vi "Main.vi"() -> ()   [LabVIEW 2018] (continued)
            n1595 = Concatenate Strings("Where QRCode='" ("查询语句"), w1146, "'" ("字符串")) -> (w1171:string)
            n1596 = call "SQL_Select.vi"("要读取的列名"=string[] ["Last_Station", "Last_Result"], "表名"="Online", "error in (no error)"=w1177, "查询语句"=w1171, "查询条件"=TRUE, "connection reference"=w1178) -> ("error out"=w1150:errorcluster, "数据"=w1170:string[][])  [unwired: 3 in, 1 out]
            n1597 = case shown="无错误" w1150 {
              tunnel: w1170 -> [w1185 _]
              tunnel: ["1" ("右扫码请求回复") "2" ("右扫码请求回复")] -> w1162
              tunnel: [w1180 w1186] -> w1161
              tunnel: [w1179 w1186] -> w1160
              frame No Error {
                n1598 = Index Array(array=w1185, index (row)=0 ("索引 (行)")) -> (element=w1182:string[])  [unwired: 1 in]
                n1599 = Index Array(array=w1182, index #1=0 ("索引 (行)")) -> (element #1=w1180:string, element #2=w1179:string)  [unwired: 1 in]
                "上一站号(102)" <- w1180
                "上一站结果(102)" <- w1179
              }
              frame Error {
                w1186 = ""
              }
            }
            n1600 = Insert Into Array(array=string[] [] ("数组"), index=0 ("索引"), new element #1=w1162, new element #2=w1161, new element #3=w1160) -> (w1167:string[])
            n1601 = Format Date/Time String(time format string (%c)="%Y-%m-%d" ("时间格式字符串(%c)")) -> (date/time string=w1158:string)  [unwired: 2 in]
            n1602 = Get Date/Time String() -> (time string=w1157:string)  [unwired: 3 in, 1 out]
            n1603 = Bundle By Name(cluster=cluster{"Data":string[], "State":T1} {"Data"=[], "State"=enum."PLC通讯初始化"} ("元素"), "Data"=w1167, "State"=状态2."扫码回复2") -> (w1168:cluster{"Data":string[], "State":T1})
            n1604 = Enqueue Element(queue=w1163, element=w1168) -> ()  [unwired: 2 in, 3 out]
            n1605 = Insert Into Array(array=string[] [] ("数组"), index=0 ("索引"), new element #1=w1158, new element #2=w1157, new element #3=w1146) -> (w1154:string[])
            n1606 = Insert Into Array(array=string[][] [] ("数组"), index (row)=0 ("索引 (行)"), new element=w1154) -> (w1151:string[][])  [unwired: 1 in]
            n1607 = Transpose 2D Array(2D array=w1151) -> (transposed array=w1148:string[][])
            n1608 = property on="ST10-2_DATA" class="MCListbox (严格)"("ItemNames"=w1148) -> ()  [unwired: 2 in, 2 out]
          }
          event "ST102数据读取（事件）": Value Change {
            w1211 = 0 ("索引 (行)")
            n1609 = event-data() -> ()  [unwired: 1 in, 2 out]
            n1610 = local read "102读取数据"() -> (w1188:string[])
            n1611 = local read "102 二维码"() -> (w1193:string)
            n1612 = Concatenate Strings("Where QRCode='" ("查询语句"), w1193, "'" ("字符串")) -> (w1218:string)
            n1613 = call "SQL_Select.vi"("要读取的列名"=string[] ["Rework_Status"], "表名"="Online", "error in (no error)"=w1195, "查询语句"=w1218, "查询条件"=TRUE, "connection reference"=w1196) -> ("error out"=w1213:errorcluster, "数据"=w1217:string[][], "connection reference out"=w1214:T12)  [unwired: 3 in]
            n1614 = Index Array(array=w1217, index (row)=w1211, index (col)=w1211) -> (element=w1216:string)
            n1615 = Equal?(x=w1216, y="T") -> (x = y?=w1215:bool)
            n1616 = case shown="真" w1215 {
              tunnel: [w1235 w1241] -> w1223
              tunnel: w1188 -> [w1234 w1244]
              tunnel: [w1229 w1240] -> w1191
              tunnel: w1193 -> [w1228 w1243]
              tunnel: w1218 -> [w1227 w1242]
              tunnel: w1214 -> [w1226 w1255]
              tunnel: w1213 -> [w1225 w1254]
              frame False {
                n1617 = call "SQL_Update.vi"("查询语句"=w1227, "表名"="Online", "error in (no error)"=w1225, "列名对应的值"=w1234, "列名"=string[] ["Last_Station", "Last_Result", "ST102_Date", "ST102_Time", "ST102_Package_Result"], "connection reference"=w1226) -> ("error out"=w1229:errorcluster)  [unwired: 4 in, 1 out]
                n1618 = Unbundle By Name(w1229) -> ("status"=w1233:bool)
                n1619 = Equal?(x=w1228, y="") -> (x = y?=w1231:bool)
                n1620 = Or(x=w1233, y=w1231) -> (x .or. y?=w1230:bool)
                n1621 = case shown="假" w1230 {
                  tunnel: ["1" ("数据保存请求回复") "2" ("数据保存请求回复")] -> w1235
                  frame False {
                  }
                  frame True {
                  }
                }
              }
              frame True {
                w1250 = 0 ("索引 (行)")
                n1622 = call "SQL_Select.vi"("要读取的列名"=string[] ["[102]"], "表名"="Rework_List", "error in (no error)"=w1254, "查询语句"=w1242, "查询条件"=TRUE, "connection reference"=w1255) -> ("error out"=w1245:errorcluster, "数据"=w1251:string[][], "connection reference out"=w1246:T12)  [unwired: 3 in]
                n1623 = Index Array(array=w1251, index (row)=w1250, index (col)=w1250) -> (element=w1249:string)
                n1624 = Equal?(x=w1249, y="T") -> (x = y?=w1247:bool)
                n1625 = case shown="真" w1247 {
                  tunnel: w1246 -> [w1263 w1282]
                  tunnel: w1245 -> [w1264 w1281]
                  tunnel: w1244 -> [w1262 w1288]
                  tunnel: w1243 -> [w1259 w1283]
                  tunnel: w1242 -> [w1261 w1275]
                  tunnel: [w1258 w1274] -> w1241
                  tunnel: [w1260 w1273] -> w1240
                  frame False {
                    n1626 = call "SQL_Update.vi"("查询语句"=w1261, "表名"="Online", "error in (no error)"=w1264, "列名对应的值"=w1262, "列名"=string[] ["Last_Station", "Last_Result", "ST101_Date", "ST101_Time", "ST101_Package_Result", "ST101_Shaft_M0102049", "ST101_Form_Seal_5026859", "ST101_Dowel_Pin_5024532", "ST101_Dowel_Pin_5020281", "ST101_Control_Plat_5025303", "ST101_Flange_M0104918"], "connection reference"=w1263) -> ("error out"=w1260:errorcluster)  [unwired: 4 in, 1 out]
                    n1627 = Unbundle By Name(w1260) -> ("status"=w1268:bool)
                    n1628 = Equal?(x=w1259, y="") -> (x = y?=w1266:bool)
                    n1629 = Or(x=w1268, y=w1266) -> (x .or. y?=w1265:bool)
                    n1630 = case shown="假" w1265 {
                      tunnel: ["1" ("数据保存请求回复") "2" ("数据保存请求回复")] -> w1258
                      frame False {
                      }
                      frame True {
                      }
                    }
                  }
                  frame True {
                    n1631 = Delete From Array(array=w1288, length=2 ("长度"), index=0 ("索引")) -> (deleted portion=w1276:string[], array with subset deleted=w1285:string[])
                    n1632 = call "SQL_Update.vi"("查询语句"=w1275, "表名"="Online", "error in (no error)"=w1281, "列名对应的值"=w1276, "列名"=string[] ["Last_Station", "Last_Result"], "connection reference"=w1282) -> ("error out"=w1280:errorcluster, "connection reference 2"=w1279:T12)  [unwired: 4 in]
                    n1633 = call "SQL_Update.vi"("查询语句"=w1275, "表名"="Rework", "error in (no error)"=w1280, "列名对应的值"=w1285, "列名"=string[] ["ST102_Date", "ST102_Time", "ST102_Package_Result"], "connection reference"=w1279) -> ("error out"=w1273:errorcluster)  [unwired: 4 in, 1 out]
                    n1634 = Unbundle By Name(w1273) -> ("status"=w1291:bool)
                    n1635 = Equal?(x="", y=w1283) -> (x = y?=w1290:bool)
                    n1636 = Or(x=w1291, y=w1290) -> (x .or. y?=w1289:bool)
                    n1637 = case shown="假" w1289 {
                      tunnel: ["1" ("数据保存请求回复") "2" ("数据保存请求回复")] -> w1274
                      frame False {
                      }
                      frame True {
                      }
                    }
                  }
                }
              }
            }
            n1638 = Insert Into Array(array=string[] [] ("数组"), index=0 ("索引"), new element=w1223) -> (w1224:string[])
            n1639 = Delete From Array(array=w1188, length=2 ("长度"), index=0 ("索引")) -> (array with subset deleted=w1220:string[])  [unwired: 1 out]
            n1640 = Bundle By Name(cluster=cluster{"Data":string[], "State":T1} {"Data"=[], "State"=enum."PLC通讯初始化"} ("元素"), "Data"=w1224, "State"=状态2."数据保存回复2") -> (w1222:cluster{"Data":string[], "State":T1})
            n1641 = Insert Into Array(array=w1220, index=2 ("索引"), new element=w1193) -> (w1219:string[])
            n1642 = Enqueue Element(queue=w1194, element=w1222) -> ()  [unwired: 2 in, 3 out]
            n1643 = Insert Into Array(array=string[][] [] ("数组"), index (row)=0 ("索引 (行)"), new element=w1219) -> (w1221:string[][])  [unwired: 1 in]
            n1644 = Transpose 2D Array(2D array=w1221) -> (transposed array=w1192:string[][])
            n1645 = property on="ST10-2_DATA" class="MCListbox (严格)"("ItemNames"=w1192) -> ()  [unwired: 2 in, 2 out]
            "ST102数据读取（事件）" <- FALSE ("ST102数据读取（事件）")
          }
          event "ST202扫码请求(事件)": Value Change {
            n1646 = event-data() -> ()  [unwired: 1 in, 1 out]
            n1647 = local read "201二维码"() -> (w1295:string)
            n1648 = Concatenate Strings("Where QRCode='" ("查询语句"), w1295, "'" ("字符串")) -> (w1321:string)
            n1649 = call "SQL_Select.vi"("要读取的列名"=string[] ["Last_Station", "Last_Result"], "表名"="Online", "error in (no error)"=w1301, "查询语句"=w1321, "查询条件"=TRUE, "connection reference"=w1300) -> ("error out"=w1297:errorcluster, "数据"=w1320:string[][])  [unwired: 3 in, 1 out]
            n1650 = case shown="无错误" w1297 {
              tunnel: w1320 -> [w1334 _]
              tunnel: ["1" ("右扫码请求回复") "2" ("右扫码请求回复")] -> w1313
              tunnel: [w1329 w1335] -> w1312
              tunnel: [w1328 w1335] -> w1311
              frame No Error {
                n1651 = Index Array(array=w1334, index (row)=0 ("索引 (行)")) -> (element=w1331:string[])  [unwired: 1 in]
                n1652 = Index Array(array=w1331, index #1=0 ("索引 (行)")) -> (element #1=w1329:string, element #2=w1328:string)  [unwired: 1 in]
                "上一站号 (202)" <- w1329
                "上一站结果 (202)" <- w1328
              }
              frame Error {
                w1335 = ""
              }
            }
            n1653 = Insert Into Array(array=string[] [] ("数组"), index=0 ("索引"), new element #1=w1313, new element #2=w1312, new element #3=w1311) -> (w1317:string[])
            n1654 = Format Date/Time String(time format string (%c)="%Y-%m-%d" ("时间格式字符串(%c)")) -> (date/time string=w1309:string)  [unwired: 2 in]
            n1655 = Get Date/Time String() -> (time string=w1308:string)  [unwired: 3 in, 1 out]
            n1656 = Bundle By Name(cluster=cluster{"Data":string[], "State":T1} {"Data"=[], "State"=enum."PLC通讯初始化"} ("元素"), "Data"=w1317, "State"=状态2."扫码回复") -> (w1318:cluster{"Data":string[], "State":T1})
            n1657 = Insert Into Array(array=string[] [] ("数组"), index=0 ("索引"), new element #1=w1309, new element #2=w1308, new element #3=w1295) -> (w1305:string[])
            n1658 = Enqueue Element(queue=w1299, element=w1318) -> ()  [unwired: 2 in, 3 out]
            n1659 = Insert Into Array(array=string[][] [] ("数组"), index (row)=0 ("索引 (行)"), new element=w1305) -> (w1302:string[][])  [unwired: 1 in]
            n1660 = Transpose 2D Array(2D array=w1302) -> (transposed array=w1298:string[][])
            n1661 = property on="ST20-2_DATA" class="MCListbox (严格)"("ItemNames"=w1298) -> ()  [unwired: 2 in, 2 out]
            "ST202扫码请求(事件)" <- FALSE ("ST20扫码请求(事件)")
          }
          event "ST202数据读取(事件)": Value Change {
            w1349 = 0 ("索引 (行)")
            n1662 = event-data() -> ()  [unwired: 1 in, 1 out]
            n1663 = local read "201二维码"() -> (w1338:string)
            n1664 = local write "ST202数据读取(事件)"(FALSE ("ST20数据读取(事件)")) -> ()
            n1665 = Dequeue Element(queue=w1369, timeout in ms (-1)=10 ("超时毫秒(-1)")) -> (element=w1339:string[])  [unwired: 1 in, 3 out]
            n1666 = Concatenate Strings("Where QRCode='" ("查询语句"), w1338, "'" ("字符串")) -> (w1351:string)
            n1667 = call "SQL_Select.vi"("要读取的列名"=string[] ["Rework_Status"], "表名"="Online", "error in (no error)"=w1342, "查询语句"=w1351, "查询条件"=TRUE, "connection reference"=w1343) -> ("error out"=w1344:errorcluster, "数据"=w1350:string[][], "connection reference out"=w1345:T12)  [unwired: 3 in]
            n1668 = Index Array(array=w1350, index (row)=w1349, index (col)=w1349) -> (element=w1348:string)
            n1669 = Equal?(x=w1348, y="T") -> (x = y?=w1346:bool)
            n1670 = case shown="真" w1346 {
              tunnel: [w1387 w1392] -> w1340
              tunnel: w1339 -> [w1376 w1395]
              tunnel: [w1382 w1391] -> w1341
              tunnel: w1338 -> [w1381 w1394]
              tunnel: w1351 -> [w1380 w1393]
              tunnel: w1345 -> [w1379 w1406]
              tunnel: w1344 -> [w1378 w1405]
              frame False {
                n1671 = call "SQL_Update.vi"("查询语句"=w1380, "表名"="Online", "error in (no error)"=w1378, "列名对应的值"=w1376, "列名"=string[] ["Last_Station", "Last_Result", "ST202_Date", "ST202_Time", "ST202_Package_Result", "ST202_Rotor_5025805", "ST202_Camring_5026187", "ST202_Dowel_Pin_M0104893"], "connection reference"=w1379) -> ("error out"=w1382:errorcluster)  [unwired: 4 in, 1 out]
                n1672 = Unbundle By Name(w1382) -> ("status"=w1386:bool)
                n1673 = Equal?(x=w1381, y="") -> (x = y?=w1384:bool)
                n1674 = Or(x=w1386, y=w1384) -> (x .or. y?=w1383:bool)
                n1675 = case shown="假" w1383 {
                  tunnel: ["1" ("数据保存请求回复") "2" ("数据保存请求回复")] -> w1387
                  frame False {
                  }
                  frame True {
                  }
                }
              }
              frame True {
                w1401 = 0 ("索引 (行)")
                n1676 = call "SQL_Select.vi"("要读取的列名"=string[] ["[202]"], "表名"="Rework_List", "error in (no error)"=w1405, "查询语句"=w1393, "查询条件"=TRUE, "connection reference"=w1406) -> ("error out"=w1396:errorcluster, "数据"=w1402:string[][], "connection reference out"=w1397:T12)  [unwired: 3 in]
                n1677 = Index Array(array=w1402, index (row)=w1401, index (col)=w1401) -> (element=w1400:string)
                n1678 = Equal?(x=w1400, y="T") -> (x = y?=w1398:bool)
                n1679 = case shown="真" w1398 {
                  tunnel: w1397 -> [w1414 w1433]
                  tunnel: w1396 -> [w1415 w1432]
                  tunnel: w1395 -> [w1413 w1439]
                  tunnel: w1394 -> [w1410 w1434]
                  tunnel: w1393 -> [w1412 w1424]
                  tunnel: [w1409 w1426] -> w1392
                  tunnel: [w1411 w1425] -> w1391
                  frame False {
                    n1680 = call "SQL_Update.vi"("查询语句"=w1412, "表名"="Online", "error in (no error)"=w1415, "列名对应的值"=w1413, "列名"=string[] ["Last_Station", "Last_Result", "ST202_Date", "ST202_Time", "ST202_Package_Result", "ST202_Rotor_5025805", "ST202_Camring_5026187", "ST202_Dowel_Pin_M0104893"], "connection reference"=w1414) -> ("error out"=w1411:errorcluster)  [unwired: 4 in, 1 out]
                    n1681 = Unbundle By Name(w1411) -> ("status"=w1419:bool)
                    n1682 = Equal?(x=w1410, y="") -> (x = y?=w1417:bool)
                    n1683 = Or(x=w1419, y=w1417) -> (x .or. y?=w1416:bool)
                    n1684 = case shown="假" w1416 {
                      tunnel: ["1" ("数据保存请求回复") "2" ("数据保存请求回复")] -> w1409
                      frame False {
                      }
                      frame True {
                      }
                    }
                  }
                  frame True {
                    n1685 = Delete From Array(array=w1439, length=2 ("长度"), index=0 ("索引")) -> (deleted portion=w1427:string[], array with subset deleted=w1436:string[])
                    n1686 = call "SQL_Update.vi"("查询语句"=w1424, "表名"="Online", "error in (no error)"=w1432, "列名对应的值"=w1427, "列名"=string[] ["Last_Station", "Last_Result"], "connection reference"=w1433) -> ("error out"=w1431:errorcluster, "connection reference 2"=w1430:T12)  [unwired: 4 in]
                    n1687 = call "SQL_Update.vi"("查询语句"=w1424, "表名"="Rework", "error in (no error)"=w1431, "列名对应的值"=w1436, "列名"=string[] ["ST202_Date", "ST202_Time", "ST202_Package_Result", "ST202_Rotor_5025805", "ST202_Camring_5026187", "ST202_Dowel_Pin_M0104893"], "connection reference"=w1430) -> ("error out"=w1425:errorcluster)  [unwired: 4 in, 1 out]
                    n1688 = Unbundle By Name(w1425) -> ("status"=w1442:bool)
                    n1689 = Equal?(x="", y=w1434) -> (x = y?=w1441:bool)
                    n1690 = Or(x=w1442, y=w1441) -> (x .or. y?=w1440:bool)
                    n1691 = case shown="真" w1440 {
                      tunnel: ["1" ("数据保存请求回复") "2" ("数据保存请求回复")] -> w1426
                      frame False {
                      }
                      frame True {
                      }
                    }
                  }
                }
              }
            }
            n1692 = Insert Into Array(array=string[] [] ("数组"), index=0 ("索引"), new element=w1340) -> (w1374:string[])
            n1693 = Bundle By Name(cluster=cluster{"Data":string[], "State":T1} {"Data"=[], "State"=enum."PLC通讯初始化"} ("元素"), "Data"=w1374, "State"=状态2."数据保存回复") -> (w1370:cluster{"Data":string[], "State":T1})
            n1694 = Delete From Array(array=w1339, length=2 ("长度"), index=0 ("索引")) -> (array with subset deleted=w1362:string[])  [unwired: 1 out]
            n1695 = Enqueue Element(queue=w1368, element=w1370) -> ()  [unwired: 2 in, 3 out]
            n1696 = Insert Into Array(array=w1362, index=2 ("索引"), new element=w1338) -> (w1360:string[])
            n1697 = Insert Into Array(array=string[][] [] ("数组"), index (row)=0 ("索引 (行)"), new element=w1360) -> (w1365:string[][])  [unwired: 1 in]
            n1698 = Transpose 2D Array(2D array=w1365) -> (transposed array=w1359:string[][])
            n1699 = property on="ST20-2_DATA" class="MCListbox (严格)"("ItemNames"=w1359) -> ()  [unwired: 2 in, 2 out]
          }
          event "ST203扫码请求（事件）": Value Change {
            n1700 = event-data() -> ()  [unwired: 1 in, 2 out]
            n1701 = local read "202二维码"() -> (w1446:string)
            n1702 = Concatenate Strings("Where QRCode='" ("查询语句"), w1446, "'" ("字符串")) -> (w1477:string)
            n1703 = call "SQL_Select.vi"("要读取的列名"=string[] ["Last_Station", "Last_Result"], "表名"="Online", "error in (no error)"=w1451, "查询语句"=w1477, "查询条件"=TRUE, "connection reference"=w1452) -> ("error out"=w1449:errorcluster, "数据"=w1476:string[][])  [unwired: 3 in, 1 out]
            n1704 = case shown="无错误" w1449 {
              tunnel: w1476 -> [w1485 _]
              tunnel: ["1" ("右扫码请求回复") "2" ("右扫码请求回复")] -> w1473
              tunnel: [w1480 w1486] -> w1472
              tunnel: [w1479 w1486] -> w1471
              frame No Error {
                n1705 = Index Array(array=w1485, index (row)=0 ("索引 (行)")) -> (element=w1482:string[])  [unwired: 1 in]
                n1706 = Index Array(array=w1482, index #1=0 ("索引 (行)")) -> (element #1=w1480:string, element #2=w1479:string)  [unwired: 1 in]
                "上一站号 (203)" <- w1480
                "上一站结果 (203)" <- w1479
              }
              frame Error {
                w1486 = ""
              }
            }
            n1707 = Insert Into Array(array=string[] [] ("数组"), index=0 ("索引"), new element #1=w1473, new element #2=w1472, new element #3=w1471) -> (w1474:string[])
            n1708 = Format Date/Time String(time format string (%c)="%Y-%m-%d" ("时间格式字符串(%c)")) -> (date/time string=w1470:string)  [unwired: 2 in]
            n1709 = Get Date/Time String() -> (time string=w1469:string)  [unwired: 3 in, 1 out]
            n1710 = Bundle By Name(cluster=cluster{"Data":string[], "State":T1} {"Data"=[], "State"=enum."PLC通讯初始化"} ("元素"), "Data"=w1474, "State"=状态2."扫码回复2") -> (w1475:cluster{"Data":string[], "State":T1})
            n1711 = Insert Into Array(array=string[] [] ("数组"), index=0 ("索引"), new element #1=w1470, new element #2=w1469, new element #3=w1446) -> (w1468:string[])
            n1712 = Enqueue Element(queue=w1450, element=w1475) -> ()  [unwired: 2 in, 3 out]
            n1713 = Insert Into Array(array=string[][] [] ("数组"), index (row)=0 ("索引 (行)"), new element=w1468) -> (w1467:string[][])  [unwired: 1 in]
            n1714 = Transpose 2D Array(2D array=w1467) -> (transposed array=w1448:string[][])
            n1715 = property on="ST20-3_DATA" class="MCListbox (严格)"("ItemNames"=w1448) -> ()  [unwired: 2 in, 2 out]
            "ST203扫码请求（事件）" <- FALSE ("ST203扫码请求（事件）")
          }
          event "ST203数据读取（事件）": Value Change {
            w1510 = 0 ("索引 (行)")
            n1716 = event-data() -> ()  [unwired: 1 in, 2 out]
            n1717 = local read "202二维码"() -> (w1492:string)
            n1718 = local read "202读取数据"() -> (w1488:string[])
            n1719 = Concatenate Strings("Where QRCode='" ("查询语句"), w1492, "'" ("字符串")) -> (w1518:string)
            n1720 = call "SQL_Select.vi"("要读取的列名"=string[] ["Rework_Status"], "表名"="Online", "error in (no error)"=w1494, "查询语句"=w1518, "查询条件"=TRUE, "connection reference"=w1495) -> ("error out"=w1513:errorcluster, "数据"=w1517:string[][], "connection reference out"=w1514:T12)  [unwired: 3 in]
            n1721 = Index Array(array=w1517, index (row)=w1510, index (col)=w1510) -> (element=w1516:string)
            n1722 = Equal?(x=w1516, y="T") -> (x = y?=w1515:bool)
            n1723 = case shown="真" w1515 {
              tunnel: [w1536 w1541] -> w1512
              tunnel: w1488 -> [w1535 w1544]
              tunnel: [w1530 w1540] -> w1490
              tunnel: w1492 -> [w1529 w1543]
              tunnel: w1518 -> [w1528 w1542]
              tunnel: w1514 -> [w1527 w1555]
              tunnel: w1513 -> [w1526 w1554]
              frame False {
                n1724 = call "SQL_Update.vi"("查询语句"=w1528, "表名"="Online", "error in (no error)"=w1526, "列名对应的值"=w1535, "列名"=string[] ["Last_Station", "Last_Result", "ST203_Date", "ST203_Time", "ST203_Package_Result", "ST203_magnetic_flux_L", "ST203_magnetic_flux_R", "ST203_magnetic_flux_Upper", "ST203_magnetic_flux_Lower"], "connection reference"=w1527) -> ("error out"=w1530:errorcluster)  [unwired: 4 in, 1 out]
                n1725 = Unbundle By Name(w1530) -> ("status"=w1534:bool)
                n1726 = Equal?(x=w1529, y="") -> (x = y?=w1532:bool)
                n1727 = Or(x=w1534, y=w1532) -> (x .or. y?=w1531:bool)
                n1728 = case shown="假" w1531 {
                  tunnel: ["1" ("数据保存请求回复") "2" ("数据保存请求回复")] -> w1536
                  frame False {
                  }
                  frame True {
                  }
                }
              }
              frame True {
                w1550 = 0 ("索引 (行)")
                n1729 = call "SQL_Select.vi"("要读取的列名"=string[] ["[203]"], "表名"="Rework_List", "error in (no error)"=w1554, "查询语句"=w1542, "查询条件"=TRUE, "connection reference"=w1555) -> ("error out"=w1545:errorcluster, "数据"=w1551:string[][], "connection reference out"=w1546:T12)  [unwired: 3 in]
                n1730 = Index Array(array=w1551, index (row)=w1550, index (col)=w1550) -> (element=w1549:string)
                n1731 = Equal?(x=w1549, y="T") -> (x = y?=w1547:bool)
                n1732 = case shown="真" w1547 {
                  tunnel: w1546 -> [w1563 w1582]
                  tunnel: w1545 -> [w1564 w1581]
                  tunnel: w1544 -> [w1562 w1588]
                  tunnel: w1543 -> [w1559 w1583]
                  tunnel: w1542 -> [w1561 w1573]
                  tunnel: [w1558 w1575] -> w1541
                  tunnel: [w1560 w1574] -> w1540
                  frame False {
                    n1733 = call "SQL_Update.vi"("查询语句"=w1561, "表名"="Online", "error in (no error)"=w1564, "列名对应的值"=w1562, "列名"=string[] ["Last_Station", "Last_Result", "ST203_Date", "ST203_Time", "ST203_Package_Result", "ST203_magnetic_flux_L", "ST203_magnetic_flux_R", "ST203_magnetic_flux_Upper", "ST203_magnetic_flux_Lower"], "connection reference"=w1563) -> ("error out"=w1560:errorcluster)  [unwired: 4 in, 1 out]
                    n1734 = Unbundle By Name(w1560) -> ("status"=w1568:bool)
                    n1735 = Equal?(x=w1559, y="") -> (x = y?=w1566:bool)
                    n1736 = Or(x=w1568, y=w1566) -> (x .or. y?=w1565:bool)
                    n1737 = case shown="假" w1565 {
                      tunnel: ["1" ("数据保存请求回复") "2" ("数据保存请求回复")] -> w1558
                      frame False {
                      }
                      frame True {
                      }
                    }
                  }
                  frame True {
                    n1738 = Delete From Array(array=w1588, length=2 ("长度"), index=0 ("索引")) -> (deleted portion=w1576:string[], array with subset deleted=w1585:string[])
                    n1739 = call "SQL_Update.vi"("查询语句"=w1573, "表名"="Online", "error in (no error)"=w1581, "列名对应的值"=w1576, "列名"=string[] ["Last_Station", "Last_Result"], "connection reference"=w1582) -> ("error out"=w1580:errorcluster, "connection reference 2"=w1579:T12)  [unwired: 4 in]
                    n1740 = call "SQL_Update.vi"("查询语句"=w1573, "表名"="Rework", "error in (no error)"=w1580, "列名对应的值"=w1585, "列名"=string[] ["ST203_Date", "ST203_Time", "ST203_Package_Result", "ST203_magnetic_flux_L", "ST203_magnetic_flux_R", "ST203_magnetic_flux_Upper", "ST203_magnetic_flux_Lower"], "connection reference"=w1579) -> ("error out"=w1574:errorcluster)  [unwired: 4 in, 1 out]
                    n1741 = Unbundle By Name(w1574) -> ("status"=w1591:bool)
                    n1742 = Equal?(x="", y=w1583) -> (x = y?=w1590:bool)
                    n1743 = Or(x=w1591, y=w1590) -> (x .or. y?=w1589:bool)
                    n1744 = case shown="真" w1589 {
                      tunnel: ["1" ("数据保存请求回复") "2" ("数据保存请求回复")] -> w1575
                      frame False {
                      }
                      frame True {
                      }
                    }
                  }
                }
              }
            }
            n1745 = Insert Into Array(array=string[] [] ("数组"), index=0 ("索引"), new element=w1512) -> (w1523:string[])
            n1746 = Bundle By Name(cluster=cluster{"Data":string[], "State":T1} {"Data"=[], "State"=enum."PLC通讯初始化"} ("元素"), "Data"=w1523, "State"=状态2."数据保存回复2") -> (w1522:cluster{"Data":string[], "State":T1})
            n1747 = Delete From Array(array=w1488, length=2 ("长度"), index=0 ("索引")) -> (array with subset deleted=w1520:string[])  [unwired: 1 out]
            n1748 = Enqueue Element(queue=w1493, element=w1522) -> ()  [unwired: 2 in, 3 out]
            n1749 = Insert Into Array(array=w1520, index=2 ("索引"), new element=w1492) -> (w1519:string[])
            n1750 = Insert Into Array(array=string[][] [] ("数组"), index (row)=0 ("索引 (行)"), new element=w1519) -> (w1521:string[][])  [unwired: 1 in]
            n1751 = Transpose 2D Array(2D array=w1521) -> (transposed array=w1491:string[][])
            n1752 = property on="ST20-3_DATA" class="MCListbox (严格)"("ItemNames"=w1491) -> ()  [unwired: 2 in, 2 out]
            "ST203数据读取（事件）" <- FALSE ("ST203数据读取（事件）")
          }
          event "ST301扫码请求 (事件)": Value Change {
            n1753 = event-data() -> ()  [unwired: 1 in, 1 out]
            n1754 = local read "301 二维码"() -> (w1595:string)
            n1755 = Concatenate Strings("Where QRCode='" ("查询语句"), w1595, "'" ("字符串")) -> (w1621:string)
            n1756 = call "SQL_Select.vi"("要读取的列名"=string[] ["Last_Station", "Last_Result"], "表名"="Online", "error in (no error)"=w1600, "查询语句"=w1621, "查询条件"=TRUE, "connection reference"=w1601) -> ("error out"=w1598:errorcluster, "数据"=w1620:string[][])  [unwired: 3 in, 1 out]
            n1757 = case shown="无错误" w1598 {
              tunnel: w1620 -> [w1634 _]
              tunnel: ["1" ("右扫码请求回复") "2" ("右扫码请求回复")] -> w1613
              tunnel: [w1629 w1635] -> w1612
              tunnel: [w1628 w1635] -> w1611
              frame No Error {
                n1758 = Index Array(array=w1634, index (row)=0 ("索引 (行)")) -> (element=w1631:string[])  [unwired: 1 in]
                n1759 = Index Array(array=w1631, index #1=0 ("索引 (行)")) -> (element #1=w1629:string, element #2=w1628:string)  [unwired: 1 in]
                "上一站号 (301)" <- w1629
                "上一站结果 (301)" <- w1628
              }
              frame Error {
                w1635 = ""
              }
            }
            n1760 = Insert Into Array(array=string[] [] ("数组"), index=0 ("索引"), new element #1=w1613, new element #2=w1612, new element #3=w1611) -> (w1617:string[])
            n1761 = Format Date/Time String(time format string (%c)="%Y-%m-%d" ("时间格式字符串(%c)")) -> (date/time string=w1609:string)  [unwired: 2 in]
            n1762 = Get Date/Time String() -> (time string=w1608:string)  [unwired: 3 in, 1 out]
            n1763 = Bundle By Name(cluster=cluster{"Data":string[], "State":T1} {"Data"=[], "State"=enum."PLC通讯初始化"} ("元素"), "Data"=w1617, "State"=状态2."扫码回复") -> (w1618:cluster{"Data":string[], "State":T1})
            n1764 = Insert Into Array(array=string[] [] ("数组"), index=0 ("索引"), new element #1=w1609, new element #2=w1608, new element #3=w1595) -> (w1605:string[])
            n1765 = Enqueue Element(queue=w1599, element=w1618) -> ()  [unwired: 2 in, 3 out]
            n1766 = Insert Into Array(array=string[][] [] ("数组"), index (row)=0 ("索引 (行)"), new element=w1605) -> (w1602:string[][])  [unwired: 1 in]
            n1767 = Transpose 2D Array(2D array=w1602) -> (transposed array=w1596:string[][])
            n1768 = property on="ST30-1_DATA" class="MCListbox (严格)"("ItemNames"=w1596) -> ()  [unwired: 2 in, 2 out]
            "ST301扫码请求 (事件)" <- FALSE ("ST30扫码请求 (事件)")
          }
          event "ST301数据读取 (事件)": Value Change {
            w1649 = 0 ("索引 (行)")
            n1769 = event-data() -> ()  [unwired: 1 in, 1 out]
            n1770 = Dequeue Element(queue=w1668, timeout in ms (-1)=10 ("超时毫秒(-1)")) -> (element=w1640:string[])  [unwired: 1 in, 3 out]
            n1771 = local read "301 二维码"() -> (w1638:string)
            n1772 = Concatenate Strings("Where QRCode='" ("查询语句"), w1638, "'" ("字符串")) -> (w1651:string)
            n1773 = call "SQL_Select.vi"("要读取的列名"=string[] ["Rework_Status"], "表名"="Online", "error in (no error)"=w1643, "查询语句"=w1651, "查询条件"=TRUE, "connection reference"=w1642) -> ("error out"=w1644:errorcluster, "数据"=w1650:string[][], "connection reference out"=w1645:T12)  [unwired: 3 in]
            n1774 = Index Array(array=w1650, index (row)=w1649, index (col)=w1649) -> (element=w1648:string)
            n1775 = Equal?(x=w1648, y="T") -> (x = y?=w1646:bool)
            n1776 = case shown="真" w1646 {
              tunnel: [w1687 w1692] -> w1641
              tunnel: w1640 -> [w1686 w1695]
              tunnel: [w1681 w1691] -> w1639
              tunnel: w1638 -> [w1680 w1694]
              tunnel: w1651 -> [w1679 w1693]
              tunnel: w1645 -> [w1678 w1706]
              tunnel: w1644 -> [w1677 w1705]
              frame False {
                n1777 = call "SQL_Update.vi"("查询语句"=w1679, "表名"="Online", "error in (no error)"=w1677, "列名对应的值"=w1686, "列名"=string[] ["Last_Station", "Last_Result", "ST301_Date", "ST301_Time", "ST301_Package_Result", "ST301_Vane_5004737", "ST301_Dowel_Pin_5024533", "ST301_Dowel_Pin_5020282"], "connection reference"=w1678) -> ("error out"=w1681:errorcluster)  [unwired: 4 in, 1 out]
                n1778 = Unbundle By Name(w1681) -> ("status"=w1685:bool)
                n1779 = Equal?(x=w1680, y="") -> (x = y?=w1683:bool)
                n1780 = Or(x=w1685, y=w1683) -> (x .or. y?=w1682:bool)
                n1781 = case shown="假" w1682 {
                  tunnel: ["1" ("数据保存请求回复") "2" ("数据保存请求回复")] -> w1687
                  frame False {
                  }
                  frame True {
                  }
                }
              }
              frame True {
                w1701 = 0 ("索引 (行)")
                n1782 = call "SQL_Select.vi"("要读取的列名"=string[] ["[301]"], "表名"="Rework_List", "error in (no error)"=w1705, "查询语句"=w1693, "查询条件"=TRUE, "connection reference"=w1706) -> ("error out"=w1696:errorcluster, "数据"=w1702:string[][], "connection reference out"=w1697:T12)  [unwired: 3 in]
                n1783 = Index Array(array=w1702, index (row)=w1701, index (col)=w1701) -> (element=w1700:string)
                n1784 = Equal?(x=w1700, y="T") -> (x = y?=w1698:bool)
                n1785 = case shown="假" w1698 {
                  tunnel: w1697 -> [w1714 w1733]
                  tunnel: w1696 -> [w1715 w1732]
                  tunnel: w1695 -> [w1713 w1739]
                  tunnel: w1694 -> [w1710 w1734]
                  tunnel: w1693 -> [w1712 w1724]
                  tunnel: [w1709 w1726] -> w1692
                  tunnel: [w1711 w1725] -> w1691
                  frame False {
                    n1786 = call "SQL_Update.vi"("查询语句"=w1712, "表名"="Online", "error in (no error)"=w1715, "列名对应的值"=w1713, "列名"=string[] ["Last_Station", "Last_Result", "ST301_Date", "ST301_Time", "ST301_Package_Result", "ST301_Vane_5004737", "ST301_Dowel_Pin_5024533", "ST301_Dowel_Pin_5020282"], "connection reference"=w1714) -> ("error out"=w1711:errorcluster)  [unwired: 4 in, 1 out]
                    n1787 = Unbundle By Name(w1711) -> ("status"=w1719:bool)
                    n1788 = Equal?(x=w1710, y="") -> (x = y?=w1717:bool)
                    n1789 = Or(x=w1719, y=w1717) -> (x .or. y?=w1716:bool)
                    n1790 = case shown="假" w1716 {
                      tunnel: ["1" ("数据保存请求回复") "2" ("数据保存请求回复")] -> w1709
                      frame False {
                      }
                      frame True {
                      }
                    }
                  }
                  frame True {
                    n1791 = Delete From Array(array=w1739, length=2 ("长度"), index=0 ("索引")) -> (deleted portion=w1727:string[], array with subset deleted=w1736:string[])
                    n1792 = call "SQL_Update.vi"("查询语句"=w1724, "表名"="Online", "error in (no error)"=w1732, "列名对应的值"=w1727, "列名"=string[] ["Last_Station", "Last_Result"], "connection reference"=w1733) -> ("error out"=w1731:errorcluster, "connection reference 2"=w1730:T12)  [unwired: 4 in]
                    n1793 = call "SQL_Update.vi"("查询语句"=w1724, "表名"="Rework", "error in (no error)"=w1731, "列名对应的值"=w1736, "列名"=string[] ["ST301_Date", "ST301_Time", "ST301_Package_Result", "ST301_Vane_5004737", "ST301_Dowel_Pin_5024533", "ST301_Dowel_Pin_5020282"], "connection reference"=w1730) -> ("error out"=w1725:errorcluster)  [unwired: 4 in, 1 out]
                    n1794 = Unbundle By Name(w1725) -> ("status"=w1742:bool)
                    n1795 = Equal?(x="", y=w1734) -> (x = y?=w1741:bool)
                    n1796 = Or(x=w1742, y=w1741) -> (x .or. y?=w1740:bool)
                    n1797 = case shown="真" w1740 {
                      tunnel: ["1" ("数据保存请求回复") "2" ("数据保存请求回复")] -> w1726
                      frame False {
                      }
                      frame True {
                      }
                    }
                  }
                }
              }
            }
            n1798 = Insert Into Array(array=string[] [] ("数组"), index=0 ("索引"), new element=w1641) -> (w1673:string[])
            n1799 = Delete From Array(array=w1640, length=2 ("长度"), index=0 ("索引")) -> (array with subset deleted=w1661:string[])  [unwired: 1 out]
            n1800 = Bundle By Name(cluster=cluster{"Data":string[], "State":T1} {"Data"=[], "State"=enum."PLC通讯初始化"} ("元素"), "Data"=w1673, "State"=状态2."数据保存回复") -> (w1669:cluster{"Data":string[], "State":T1})
            n1801 = Insert Into Array(array=w1661, index=2 ("索引"), new element=w1638) -> (w1659:string[])
            n1802 = Enqueue Element(queue=w1667, element=w1669) -> ()  [unwired: 2 in, 3 out]
            n1803 = Insert Into Array(array=string[][] [] ("数组"), index (row)=0 ("索引 (行)"), new element=w1659) -> (w1664:string[][])  [unwired: 1 in]
            n1804 = Transpose 2D Array(2D array=w1664) -> (transposed array=w1637:string[][])
            n1805 = property on="ST30-1_DATA" class="MCListbox (严格)"("ItemNames"=w1637) -> ()  [unwired: 2 in, 2 out]
            "ST301数据读取 (事件)" <- FALSE ("ST30数据读取 (事件)")
          }
          event "ST302扫码请求 (事件)": Value Change {
            n1806 = event-data() -> ()  [unwired: 1 in, 2 out]
            n1807 = local read "302 二维码"() -> (w1746:string)
            n1808 = Concatenate Strings("Where QRCode='" ("查询语句"), w1746, "'" ("字符串")) -> (w1777:string)
            n1809 = call "SQL_Select.vi"("要读取的列名"=string[] ["Last_Station", "Last_Result"], "表名"="Online", "error in (no error)"=w1751, "查询语句"=w1777, "查询条件"=TRUE, "connection reference"=w1752) -> ("error out"=w1749:errorcluster, "数据"=w1776:string[][])  [unwired: 3 in, 1 out]
            n1810 = case shown="无错误" w1749 {
              tunnel: w1776 -> [w1785 _]
              tunnel: ["1" ("右扫码请求回复") "2" ("右扫码请求回复")] -> w1773
              tunnel: [w1780 w1786] -> w1772
              tunnel: [w1779 w1786] -> w1771
              frame No Error {
                n1811 = Index Array(array=w1785, index (row)=0 ("索引 (行)")) -> (element=w1782:string[])  [unwired: 1 in]
                n1812 = Index Array(array=w1782, index #1=0 ("索引 (行)")) -> (element #1=w1780:string, element #2=w1779:string)  [unwired: 1 in]
                "上一站号 (302)" <- w1780
                "上一站结果 (302)" <- w1779
              }
              frame Error {
                w1786 = ""
              }
            }
            n1813 = Insert Into Array(array=string[] [] ("数组"), index=0 ("索引"), new element #1=w1773, new element #2=w1772, new element #3=w1771) -> (w1774:string[])
            n1814 = Format Date/Time String(time format string (%c)="%Y-%m-%d" ("时间格式字符串(%c)")) -> (date/time string=w1770:string)  [unwired: 2 in]
            n1815 = Get Date/Time String() -> (time string=w1769:string)  [unwired: 3 in, 1 out]
            n1816 = Bundle By Name(cluster=cluster{"Data":string[], "State":T1} {"Data"=[], "State"=enum."PLC通讯初始化"} ("元素"), "Data"=w1774, "State"=状态2."扫码回复2") -> (w1775:cluster{"Data":string[], "State":T1})
            n1817 = Insert Into Array(array=string[] [] ("数组"), index=0 ("索引"), new element #1=w1770, new element #2=w1769, new element #3=w1746) -> (w1768:string[])
            n1818 = Enqueue Element(queue=w1750, element=w1775) -> ()  [unwired: 2 in, 3 out]
            n1819 = Insert Into Array(array=string[][] [] ("数组"), index (row)=0 ("索引 (行)"), new element=w1768) -> (w1767:string[][])  [unwired: 1 in]
            n1820 = Transpose 2D Array(2D array=w1767) -> (transposed array=w1747:string[][])
            n1821 = property on="ST30-2_DATA" class="MCListbox (严格)"("ItemNames"=w1747) -> ()  [unwired: 2 in, 2 out]
            "ST302扫码请求 (事件)" <- FALSE ("ST302扫码请求 (事件)")
          }
          event "ST302数据读取 (事件)": Value Change {
            w1810 = 0 ("索引 (行)")
            n1822 = event-data() -> ()  [unwired: 1 in, 2 out]
            n1823 = local read "302 二维码"() -> (w1790:string)
            n1824 = Concatenate Strings("Where QRCode='" ("查询语句"), w1790, "'" ("字符串")) -> (w1818:string)
            n1825 = local read "302读取数据"() -> (w1788:string[])
            n1826 = call "SQL_Select.vi"("要读取的列名"=string[] ["Rework_Status"], "表名"="Online", "error in (no error)"=w1794, "查询语句"=w1818, "查询条件"=TRUE, "connection reference"=w1795) -> ("error out"=w1813:errorcluster, "数据"=w1817:string[][], "connection reference out"=w1814:T12)  [unwired: 3 in]
            n1827 = Index Array(array=w1817, index (row)=w1810, index (col)=w1810) -> (element=w1816:string)
            n1828 = Equal?(x=w1816, y="T") -> (x = y?=w1815:bool)
            n1829 = case shown="真" w1815 {
              tunnel: [w1836 w1841] -> w1812
              tunnel: w1788 -> [w1835 w1844]
              tunnel: [w1830 w1840] -> w1792
              tunnel: w1790 -> [w1829 w1843]
              tunnel: w1818 -> [w1828 w1842]
              tunnel: w1814 -> [w1827 w1855]
              tunnel: w1813 -> [w1826 w1854]
              frame False {
                n1830 = call "SQL_Update.vi"("查询语句"=w1828, "表名"="Online", "error in (no error)"=w1826, "列名对应的值"=w1835, "列名"=string[] ["Last_Station", "Last_Result", "ST302_Date", "ST302_Time", "ST302_Package_Result", "ST302_Thin_PIN_Data", "ST302_Coarse_PIN_Data", "ST302_Thin_PIN_Tolerance", "ST302_Coarse_PIN_Tolerance"], "connection reference"=w1827) -> ("error out"=w1830:errorcluster)  [unwired: 4 in, 1 out]
                n1831 = Unbundle By Name(w1830) -> ("status"=w1834:bool)
                n1832 = Equal?(x=w1829, y="") -> (x = y?=w1832:bool)
                n1833 = Or(x=w1834, y=w1832) -> (x .or. y?=w1831:bool)
                n1834 = case shown="假" w1831 {
                  tunnel: ["1" ("数据保存请求回复") "2" ("数据保存请求回复")] -> w1836
                  frame False {
                  }
                  frame True {
                  }
                }
              }
              frame True {
                w1850 = 0 ("索引 (行)")
                n1835 = call "SQL_Select.vi"("要读取的列名"=string[] ["[302]"], "表名"="Rework_List", "error in (no error)"=w1854, "查询语句"=w1842, "查询条件"=TRUE, "connection reference"=w1855) -> ("error out"=w1845:errorcluster, "数据"=w1851:string[][], "connection reference out"=w1846:T12)  [unwired: 3 in]
                n1836 = Index Array(array=w1851, index (row)=w1850, index (col)=w1850) -> (element=w1849:string)
                n1837 = Equal?(x=w1849, y="T") -> (x = y?=w1847:bool)
                n1838 = case shown="假" w1847 {
                  tunnel: w1846 -> [w1863 w1882]
                  tunnel: w1845 -> [w1864 w1881]
                  tunnel: w1844 -> [w1862 w1888]
                  tunnel: w1843 -> [w1859 w1883]
                  tunnel: w1842 -> [w1861 w1873]
                  tunnel: [w1858 w1875] -> w1841
                  tunnel: [w1860 w1874] -> w1840
                  frame False {
                    n1839 = call "SQL_Update.vi"("查询语句"=w1861, "表名"="Online", "error in (no error)"=w1864, "列名对应的值"=w1862, "列名"=string[] ["Last_Station", "Last_Result", "ST302_Date", "ST302_Time", "ST302_Package_Result", "ST302_Thin_PIN_Data", "ST302_Coarse_PIN_Data", "ST302_Thin_PIN_Tolerance", "ST302_Coarse_PIN_Tolerance"], "connection reference"=w1863) -> ("error out"=w1860:errorcluster)  [unwired: 4 in, 1 out]
                    n1840 = Unbundle By Name(w1860) -> ("status"=w1868:bool)
                    n1841 = Equal?(x=w1859, y="") -> (x = y?=w1866:bool)
                    n1842 = Or(x=w1868, y=w1866) -> (x .or. y?=w1865:bool)
                    n1843 = case shown="假" w1865 {
                      tunnel: ["1" ("数据保存请求回复") "2" ("数据保存请求回复")] -> w1858
                      frame False {
                      }
                      frame True {
                      }
                    }
                  }
                  frame True {
                    n1844 = Delete From Array(array=w1888, length=2 ("长度"), index=0 ("索引")) -> (deleted portion=w1876:string[], array with subset deleted=w1885:string[])
                    n1845 = call "SQL_Update.vi"("查询语句"=w1873, "表名"="Online", "error in (no error)"=w1881, "列名对应的值"=w1876, "列名"=string[] ["Last_Station", "Last_Result"], "connection reference"=w1882) -> ("error out"=w1880:errorcluster, "connection reference 2"=w1879:T12)  [unwired: 4 in]
                    n1846 = call "SQL_Update.vi"("查询语句"=w1873, "表名"="Rework", "error in (no error)"=w1880, "列名对应的值"=w1885, "列名"=string[] ["ST302_Date", "ST302_Time", "ST302_Package_Result", "ST302_Thin_PIN_Data", "ST302_Coarse_PIN_Data", "ST302_Thin_PIN_Tolerance", "ST302_Coarse_PIN_Tolerance"], "connection reference"=w1879) -> ("error out"=w1874:errorcluster)  [unwired: 4 in, 1 out]
                    n1847 = Unbundle By Name(w1874) -> ("status"=w1891:bool)
                    n1848 = Equal?(x="", y=w1883) -> (x = y?=w1890:bool)
                    n1849 = Or(x=w1891, y=w1890) -> (x .or. y?=w1889:bool)
                    n1850 = case shown="真" w1889 {
                      tunnel: ["1" ("数据保存请求回复") "2" ("数据保存请求回复")] -> w1875
                      frame False {
                      }
                      frame True {
                      }
                    }
                  }
                }
              }
            }
            n1851 = Insert Into Array(array=string[] [] ("数组"), index=0 ("索引"), new element=w1812) -> (w1823:string[])
            n1852 = Delete From Array(array=w1788, length=2 ("长度"), index=0 ("索引")) -> (array with subset deleted=w1820:string[])  [unwired: 1 out]
            n1853 = Bundle By Name(cluster=cluster{"Data":string[], "State":T1} {"Data"=[], "State"=enum."PLC通讯初始化"} ("元素"), "Data"=w1823, "State"=状态2."数据保存回复2") -> (w1822:cluster{"Data":string[], "State":T1})
            n1854 = Insert Into Array(array=w1820, index=2 ("索引"), new element=w1790) -> (w1819:string[])
            n1855 = Enqueue Element(queue=w1793, element=w1822) -> ()  [unwired: 2 in, 3 out]
            n1856 = Insert Into Array(array=string[][] [] ("数组"), index (row)=0 ("索引 (行)"), new element=w1819) -> (w1821:string[][])  [unwired: 1 in]
            n1857 = Transpose 2D Array(2D array=w1821) -> (transposed array=w1789:string[][])
            n1858 = property on="ST30-2_DATA" class="MCListbox (严格)"("ItemNames"=w1789) -> ()  [unwired: 2 in, 2 out]
            "ST302数据读取 (事件)" <- FALSE ("ST302数据读取 (事件)")
          }
          event "ST401扫码请求(事件)": Value Change {
            n1859 = event-data() -> ()  [unwired: 1 in, 1 out]
            n1860 = local read "401二维码"() -> (w1895:string)
            n1861 = Concatenate Strings("Where QRCode='" ("查询语句"), w1895, "'" ("字符串")) -> (w1899:string)
            n1862 = call "SQL_Select.vi"("要读取的列名"=string[] ["Last_Station", "Last_Result"], "表名"="Online", "error in (no error)"=w1897, "查询语句"=w1899, "查询条件"=TRUE, "connection reference"=w1898) -> ("error out"=w1901:errorcluster, "数据"=w1921:string[][])  [unwired: 3 in, 1 out]
            n1863 = case shown="无错误" w1901 {
              tunnel: w1921 -> [w1934 _]
              tunnel: ["1" ("右扫码请求回复") "2" ("右扫码请求回复")] -> w1914
              tunnel: [w1931 w1935] -> w1913
              tunnel: [w1930 w1935] -> w1912
              frame No Error {
                n1864 = Index Array(array=w1934, index (row)=0 ("索引 (行)")) -> (element=w1929:string[])  [unwired: 1 in]
                n1865 = Index Array(array=w1929, index #1=0 ("索引 (行)")) -> (element #1=w1931:string, element #2=w1930:string)  [unwired: 1 in]
                "上一站号 (401)" <- w1931
                "上一站结果 (401)" <- w1930
              }
              frame Error {
                w1935 = ""
              }
            }
            n1866 = Insert Into Array(array=string[] [] ("数组"), index=0 ("索引"), new element #1=w1914, new element #2=w1913, new element #3=w1912) -> (w1918:string[])
            n1867 = Format Date/Time String(time format string (%c)="%Y-%m-%d" ("时间格式字符串(%c)")) -> (date/time string=w1910:string)  [unwired: 2 in]
            n1868 = Get Date/Time String() -> (time string=w1909:string)  [unwired: 3 in, 1 out]
            n1869 = Bundle By Name(cluster=cluster{"Data":string[], "State":T1} {"Data"=[], "State"=enum."PLC通讯初始化"} ("元素"), "Data"=w1918, "State"=状态2."扫码回复") -> (w1919:cluster{"Data":string[], "State":T1})
            n1870 = Insert Into Array(array=string[] [] ("数组"), index=0 ("索引"), new element #1=w1910, new element #2=w1909, new element #3=w1895) -> (w1906:string[])
            n1871 = Enqueue Element(queue=w1902, element=w1919) -> ()  [unwired: 2 in, 3 out]
            n1872 = Insert Into Array(array=string[][] [] ("数组"), index (row)=0 ("索引 (行)"), new element=w1906) -> (w1903:string[][])  [unwired: 1 in]
            n1873 = Transpose 2D Array(2D array=w1903) -> (transposed array=w1896:string[][])
            n1874 = property on="ST40-1_DATA" class="MCListbox (严格)"("ItemNames"=w1896) -> ()  [unwired: 2 in, 2 out]
            "ST401扫码请求(事件)" <- FALSE ("ST40扫码请求(事件)")
          }
          event "ST401数据读取（事件）": Value Change {
            w1950 = 0 ("索引 (行)")
            n1875 = event-data() -> ()  [unwired: 1 in, 1 out]
            n1876 = Dequeue Element(queue=w1968, timeout in ms (-1)=10 ("超时毫秒(-1)")) -> (element=w1943:string[])  [unwired: 1 in, 3 out]
            n1877 = local read "401二维码"() -> (w1938:string)
            n1878 = Concatenate Strings("Where QRCode='" ("查询语句"), w1938, "'" ("字符串")) -> (w1941:string)
            n1879 = call "SQL_Select.vi"("要读取的列名"=string[] ["Rework_Status"], "表名"="Online", "error in (no error)"=w1939, "查询语句"=w1941, "查询条件"=TRUE, "connection reference"=w1940) -> ("error out"=w1945:errorcluster, "数据"=w1951:string[][], "connection reference out"=w1946:T12)  [unwired: 3 in]
            n1880 = Index Array(array=w1951, index (row)=w1950, index (col)=w1950) -> (element=w1949:string)
            n1881 = Equal?(x=w1949, y="T") -> (x = y?=w1947:bool)
            n1882 = case shown="假" w1947 {
              tunnel: [w1987 w1992] -> w1944
              tunnel: w1943 -> [w1986 w1995]
              tunnel: [w1981 w1991] -> w1942
              tunnel: w1938 -> [w1980 w1994]
              tunnel: w1941 -> [w1979 w1993]
              tunnel: w1946 -> [w1978 w2006]
              tunnel: w1945 -> [w1977 w2005]
              frame False {
                n1883 = call "SQL_Update.vi"("查询语句"=w1979, "表名"="Online", "error in (no error)"=w1977, "列名对应的值"=w1986, "列名"=string[] ["Last_Station", "Last_Result", "ST401_Date", "ST401_Time", "ST401_Package_Result", "ST401_Camera_Shield"], "connection reference"=w1978) -> ("error out"=w1981:errorcluster)  [unwired: 4 in, 1 out]
                n1884 = Unbundle By Name(w1981) -> ("status"=w1985:bool)
                n1885 = Equal?(x=w1980, y="") -> (x = y?=w1983:bool)
                n1886 = Or(x=w1985, y=w1983) -> (x .or. y?=w1982:bool)
                n1887 = case shown="假" w1982 {
                  tunnel: ["1" ("数据保存请求回复") "2" ("数据保存请求回复")] -> w1987
                  frame False {
                  }
                  frame True {
                  }
                }
              }
              frame True {
                w2001 = 0 ("索引 (行)")
                n1888 = call "SQL_Select.vi"("要读取的列名"=string[] ["[401]"], "表名"="Rework_List", "error in (no error)"=w2005, "查询语句"=w1993, "查询条件"=TRUE, "connection reference"=w2006) -> ("error out"=w1996:errorcluster, "数据"=w2002:string[][], "connection reference out"=w1997:T12)  [unwired: 3 in]
                n1889 = Index Array(array=w2002, index (row)=w2001, index (col)=w2001) -> (element=w2000:string)
                n1890 = Equal?(x=w2000, y="T") -> (x = y?=w1998:bool)
                n1891 = case shown="真" w1998 {
                  tunnel: w1997 -> [w2014 w2033]
                  tunnel: w1996 -> [w2015 w2032]
                  tunnel: w1995 -> [w2013 w2039]
                  tunnel: w1994 -> [w2010 w2034]
                  tunnel: w1993 -> [w2012 w2024]
                  tunnel: [w2009 w2026] -> w1992
                  tunnel: [w2011 w2025] -> w1991
                  frame False {
                    n1892 = call "SQL_Update.vi"("查询语句"=w2012, "表名"="Online", "error in (no error)"=w2015, "列名对应的值"=w2013, "列名"=string[] ["Last_Station", "Last_Result", "ST401_Date", "ST401_Time", "ST401_Package_Result", "ST401_Camera_Shield"], "connection reference"=w2014) -> ("error out"=w2011:errorcluster)  [unwired: 4 in, 1 out]
                    n1893 = Unbundle By Name(w2011) -> ("status"=w2019:bool)
                    n1894 = Equal?(x=w2010, y="") -> (x = y?=w2017:bool)
                    n1895 = Or(x=w2019, y=w2017) -> (x .or. y?=w2016:bool)
                    n1896 = case shown="假" w2016 {
                      tunnel: ["1" ("数据保存请求回复") "2" ("数据保存请求回复")] -> w2009
                      frame False {
                      }
                      frame True {
                      }
                    }
                  }
                  frame True {
                    n1897 = Delete From Array(array=w2039, length=2 ("长度"), index=0 ("索引")) -> (deleted portion=w2027:string[], array with subset deleted=w2036:string[])
                    n1898 = call "SQL_Update.vi"("查询语句"=w2024, "表名"="Online", "error in (no error)"=w2032, "列名对应的值"=w2027, "列名"=string[] ["Last_Station", "Last_Result"], "connection reference"=w2033) -> ("error out"=w2031:errorcluster, "connection reference 2"=w2030:T12)  [unwired: 4 in]
                    n1899 = call "SQL_Update.vi"("查询语句"=w2024, "表名"="Rework", "error in (no error)"=w2031, "列名对应的值"=w2036, "列名"=string[] ["ST401_Date", "ST401_Time", "ST401_Package_Result", "ST401_Camera_Shield"], "connection reference"=w2030) -> ("error out"=w2025:errorcluster)  [unwired: 4 in, 1 out]
                    n1900 = Unbundle By Name(w2025) -> ("status"=w2042:bool)
                    n1901 = Equal?(x="", y=w2034) -> (x = y?=w2041:bool)
                    n1902 = Or(x=w2042, y=w2041) -> (x .or. y?=w2040:bool)
                    n1903 = case shown="真" w2040 {
                      tunnel: ["1" ("数据保存请求回复") "2" ("数据保存请求回复")] -> w2026
                      frame False {
                      }
                      frame True {
                      }
                    }
                  }
                }
              }
            }
            n1904 = Delete From Array(array=w1943, length=2 ("长度"), index=0 ("索引")) -> (array with subset deleted=w1961:string[])  [unwired: 1 out]
            n1905 = Insert Into Array(array=string[] [] ("数组"), index=0 ("索引"), new element=w1944) -> (w1973:string[])
            n1906 = Insert Into Array(array=w1961, index=2 ("索引"), new element=w1938) -> (w1959:string[])
            n1907 = Bundle By Name(cluster=cluster{"Data":string[], "State":T1} {"Data"=[], "State"=enum."PLC通讯初始化"} ("元素"), "Data"=w1973, "State"=状态2."数据保存回复") -> (w1969:cluster{"Data":string[], "State":T1})
            n1908 = Insert Into Array(array=string[][] [] ("数组"), index (row)=0 ("索引 (行)"), new element=w1959) -> (w1964:string[][])  [unwired: 1 in]
            n1909 = Enqueue Element(queue=w1967, element=w1969) -> ()  [unwired: 2 in, 3 out]
            n1910 = Transpose 2D Array(2D array=w1964) -> (transposed array=w1937:string[][])
            n1911 = property on="ST40-1_DATA" class="MCListbox (严格)"("ItemNames"=w1937) -> ()  [unwired: 2 in, 2 out]
            "ST401数据读取（事件）" <- FALSE ("ST40数据读取（事件）")
          }
          event "ST403扫码请求(事件)": Value Change {
            n1912 = event-data() -> ()  [unwired: 1 in, 2 out]
            n1913 = local read "403二维码"() -> (w2046:string)
            n1914 = Concatenate Strings("Where QRCode='" ("查询语句"), w2046, "'" ("字符串")) -> (w2067:string)
            n1915 = call "SQL_Select.vi"("要读取的列名"=string[] ["Last_Station", "Last_Result"], "表名"="Online", "error in (no error)"=w2051, "查询语句"=w2067, "查询条件"=TRUE, "connection reference"=w2052) -> ("error out"=w2049:errorcluster, "数据"=w2077:string[][])  [unwired: 3 in, 1 out]
            n1916 = case shown="无错误" w2049 {
              tunnel: w2077 -> [w2085 _]
              tunnel: ["1" ("右扫码请求回复") "2" ("右扫码请求回复")] -> w2074
              tunnel: [w2082 w2086] -> w2073
              tunnel: [w2081 w2086] -> w2072
              frame No Error {
                n1917 = Index Array(array=w2085, index (row)=0 ("索引 (行)")) -> (element=w2080:string[])  [unwired: 1 in]
                n1918 = Index Array(array=w2080, index #1=0 ("索引 (行)")) -> (element #1=w2082:string, element #2=w2081:string)  [unwired: 1 in]
                "上一站号 (403)" <- w2082
                "上一站结果 (403)" <- w2081
              }
              frame Error {
                w2086 = ""
              }
            }
            n1919 = Format Date/Time String(time format string (%c)="%Y-%m-%d" ("时间格式字符串(%c)")) -> (date/time string=w2071:string)  [unwired: 2 in]
            n1920 = Get Date/Time String() -> (time string=w2070:string)  [unwired: 3 in, 1 out]
            n1921 = Insert Into Array(array=string[] [] ("数组"), index=0 ("索引"), new element #1=w2074, new element #2=w2073, new element #3=w2072) -> (w2075:string[])
            n1922 = Bundle By Name(cluster=cluster{"Data":string[], "State":T1} {"Data"=[], "State"=enum."PLC通讯初始化"} ("元素"), "Data"=w2075, "State"=状态2."扫码回复3") -> (w2076:cluster{"Data":string[], "State":T1})
            n1923 = Insert Into Array(array=string[] [] ("数组"), index=0 ("索引"), new element #1=w2071, new element #2=w2070, new element #3=w2046) -> (w2069:string[])
            n1924 = Enqueue Element(queue=w2050, element=w2076) -> ()  [unwired: 2 in, 3 out]
            n1925 = Insert Into Array(array=string[][] [] ("数组"), index (row)=0 ("索引 (行)"), new element=w2069) -> (w2068:string[][])  [unwired: 1 in]
            n1926 = Transpose 2D Array(2D array=w2068) -> (transposed array=w2048:string[][])
            n1927 = property on="ST40-3_DATA" class="MCListbox (严格)"("ItemNames"=w2048) -> ()  [unwired: 2 in, 2 out]
            "ST403扫码请求(事件)" <- FALSE ("ST403扫码请求(事件)")
          }
          event "ST403数据读取（事件）": Value Change {
            w2110 = 0 ("索引 (行)")
            n1928 = event-data() -> ()  [unwired: 1 in, 2 out]
            n1929 = local read "403读取数据"() -> (w2088:string[])
            n1930 = local read "403二维码"() -> (w2092:string)
            n1931 = Concatenate Strings("Where QRCode='" ("查询语句"), w2092, "'" ("字符串")) -> (w2112:string)
            n1932 = call "SQL_Select.vi"("要读取的列名"=string[] ["Rework_Status"], "表名"="Online", "error in (no error)"=w2094, "查询语句"=w2112, "查询条件"=TRUE, "connection reference"=w2095) -> ("error out"=w2114:errorcluster, "数据"=w2118:string[][], "connection reference out"=w2115:T12)  [unwired: 3 in]
            n1933 = Index Array(array=w2118, index (row)=w2110, index (col)=w2110) -> (element=w2117:string)
            n1934 = Equal?(x=w2117, y="T") -> (x = y?=w2116:bool)
            n1935 = case shown="假" w2116 {
              tunnel: [w2136 w2141] -> w2113
              tunnel: w2088 -> [w2135 w2144]
              tunnel: [w2130 w2140] -> w2090
              tunnel: w2092 -> [w2129 w2143]
